vi "BootSequenceDeviceCheck.vi"(0 "Cluster 2":T2, 5 "error out 2":errorcluster) -> (19 "error out":errorcluster)   [LabVIEW 2011]
uses:
  Utilities/controls/ctlSeqFNs_Scanner.ctl
  Utilities/controls/ctlSeqFNs_Andor.ctl
  Utilities/controls/ctlSeqFNs_CTIOTF.ctl
  Utilities/controls/ctlSeqFNs_Koheras.ctl
  Utilities/controls/ctlSeqFNs_PCDeviceInit.ctl
  Utilities/controls/ctlSeqFNs_AVTGuppy.ctl
  <vilib>/userDefined/High Color/IMAQdx.ctl
  Utilities/controls/ctlSeqFNs_Main.ctl
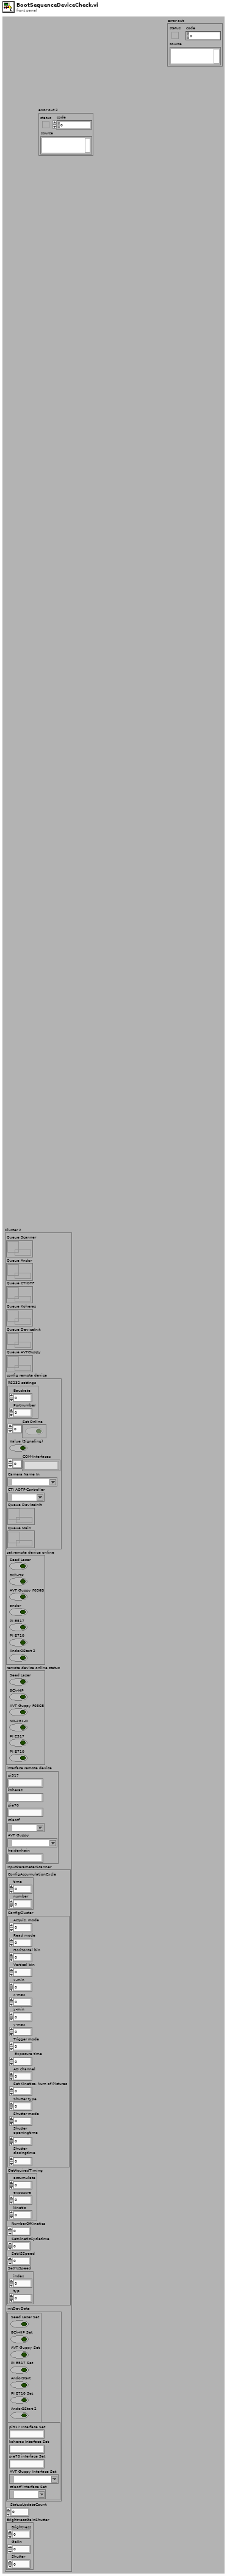
[diagram p1: front panel]
types:
  T1 = typedef "IMAQdx.ctl" = refnum<k21>
  T2 = cluster{"Queue Scanner":refnum<queue>, "Queue Andor":refnum<queue>, "Queue CTIOTF":refnum<queue>, "Queue Koheras":refnum<queue>, "Queue DeviceInit":refnum<queue>, "Queue AVTGuppy":refnum<queue>, "config remote device":cluster{"RS232 settings":cluster{"Baudrate":u16, "Portnumber":i32}, "Set Online":bool[], "Value (Signaling)":bool, "COM-Interfaces":string[], "Camera Name In":T1, "CTI AOTF-Controller":refnum<visa-resource-name>, "Queue DeviceInit":refnum<queue>, "Queue Main":refnum<queue>}, "set remote device online":cluster{"Seed Laser":bool, "8Ch-HP":bool, "AVT Guppy F036B":bool, "andor":bool, "PI E517":bool, "PI E710":bool, "Andor2Start 2":bool}, "remote device online status":cluster{"Seed Laser":bool, "8Ch-HP":bool, "AVT Guppy F036B":bool, "ND-281-D":bool, "PI E517":bool, "PI E710":bool}, "interface remote device":cluster{"pi517":string, "koheras":string, "pie70":string, "ctiaotf":refnum<visa-resource-name>, "AVT Guppy":T1, "heidenhain":string}, "InputParameterScanner":cluster{"ConfigAccumulationCycle":cluster{"time":sgl, "number":i32}, "ConfigCluster":cluster{"Acquis. mode":u16, "Read mode":u16, "Horizontal bin":i32, "Vertical bin":i32, "x-min":i32, "x-max":i32, "y-min":i32, "y-max":i32, "Trigger mode":u16, " Exposure time":sgl, "AD channel":i32, "Set Kinetics, Num of Pictures":i32, "Shutter type":u16, "Shutter mode":u16, "Shutter\nopeningtime":i32, "Shutter\nclosingtime":i32}, "GetAquiredTiming":cluster{"accumulate":sgl, "exposure":sgl, "kinetic":sgl}, "NumberOfKinetics":i32, "SetKineticCycletime":sgl, "SetVSSpeed":i32, "SetHsSpeed":cluster{"index":i32, "typ":i32}}, "initDevData":cluster{cluster{"Seed Laser Set":bool, "8Ch-HP Set":bool, "AVT Guppy Set":bool, "PI E517 Set":bool, "AndorStart":bool, "PI E710 Set":bool, "Andor2Start 2":bool}, cluster{"pi517 Interface Set":string, "koheras Interface Set":string, "pie70 interface Set":string, "AVT Guppy Interface Set":T1, "ctiaotf interface Set":refnum<visa-resource-name>}}, "StatusUpdateCount":dbl, "BrightnessGainShutter":cluster{"Brightness":i32, "Gaiin":i32, "Shutter":i32}}
  T3 = typedef "ctlSeqFNs_PCDeviceInit.ctl" = enum16{"ERROR", "INIT", "ErrorDevice", "StartDevice", "DeviceStatus", "StopDevice", "EXIT", "IDLE"}
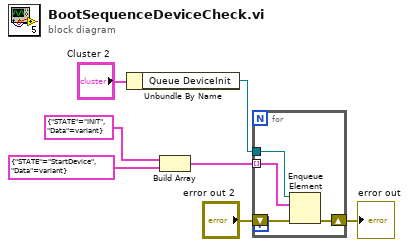
[diagram p0: block diagram]
diagram:
  n1 = Unbundle By Name("Cluster 2") -> ("Queue DeviceInit"=w4:refnum<queue>)
  n2 = Build Array(cluster{"STATE":T3, "Data":variant} {"STATE"=enum."INIT", "Data"=variant} ("element"), cluster{"STATE":T3, "Data":variant} {"STATE"=enum."StartDevice", "Data"=variant} ("element")) -> (w7:cluster{"STATE":T3, "Data":variant}[])
  n3 = for {
    tunnel: w4 -> [w11]
    tunnel: w7 -> [w10] mode=indexing
    shift-right: [w9] -> w3
    shift-left: "error out 2" -> [w8]
    n4 = Enqueue Element(queue=w11, element=w10, error in (no error)=w8) -> (error out=w9:errorcluster)  [unwired: 1 in, 2 out]
  }
  "error out" <- w3
